vi "comm control.vi"(4 "xoff character":u8, 5 "xoff limit":u16, 6 "xon character":u8, 7 "xon limit":u16, 8 "error in (no error)":errorcluster, 9 "error character":u8, 10 "flags":u32 format="%.0x", 11 "Comm Handle":u64) -> (0 "error out":errorcluster, 3 "dup Comm Handle":u64)   [LabVIEW 2009, in "lvserial.lvlib"]
doc: "Extended flow and error handling control configuration."
uses:
  lvserial.lvlib
  x64/Release/lvserial.dll
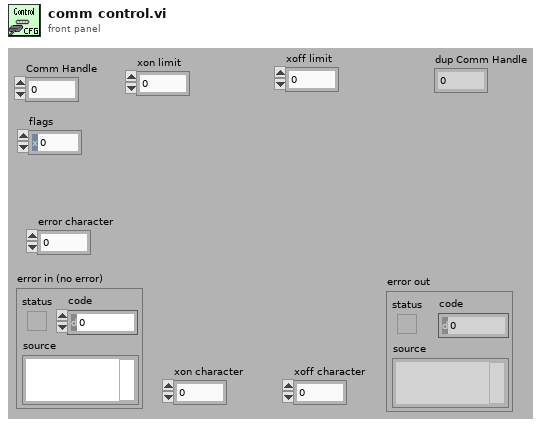
[diagram p1: front panel]
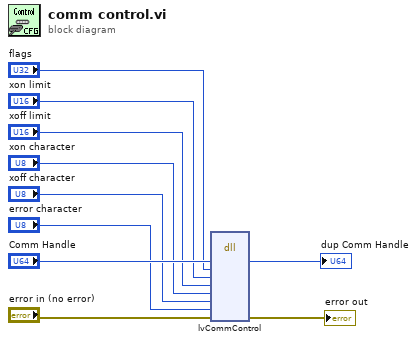
[diagram p0: block diagram]
diagram:
  n1 = dll-call lib="C:/Users/Admin/Desktop/lvserial_source_1-2-13/x64/Release/lvserial.dll" fn="lvCommControl"("hComm"="Comm Handle", "ulFlags"="flags", "usXonLim"="xon limit", "usXoffLim"="xoff limit", "cXonChar"="xon character", "cXoffChar"="xoff character", "cErrorChar"="error character", "pError"="error in (no error)") -> ("hComm"=→"dup Comm Handle":u64, "pError"=→"error out":errorcluster)  [unwired: 9 in, 3 out]
